vi "CalculateAngle_noDIO_annotated.vi"(8 "dc":dbl, 9 "Robot Beta":dbl, 10 "Robot Alpha":dbl, 11 "Beacon Theta":dbl) -> (0 "Y Position":dbl, 3 "X Position":dbl)   [LabVIEW 2014]
panel:
  out "d1":dbl
  out "K":dbl
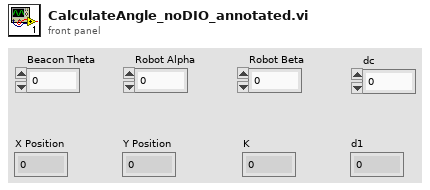
[diagram p1: front panel]
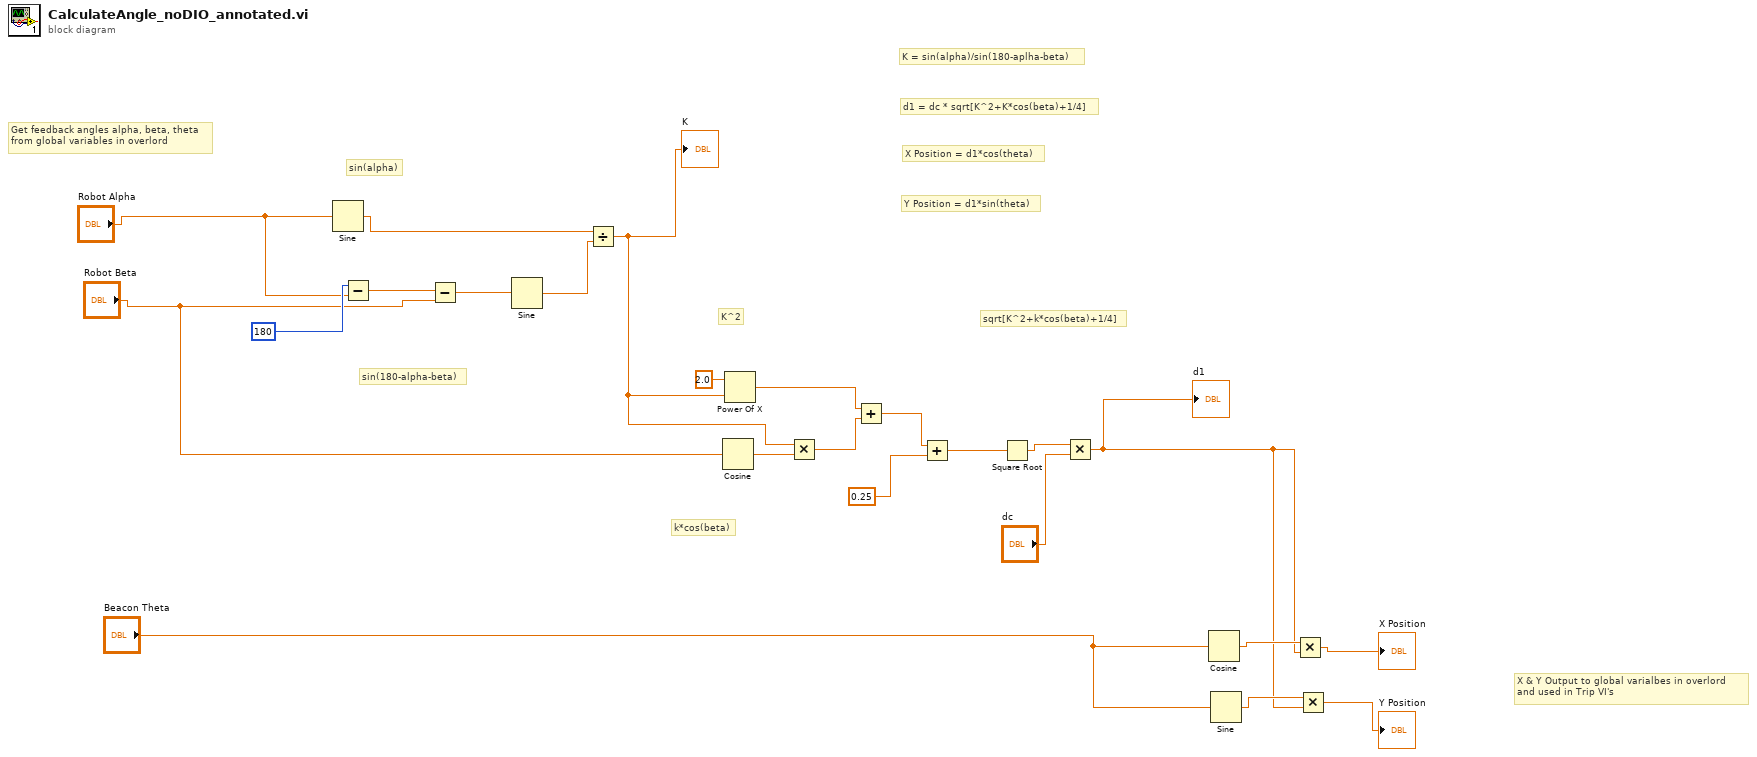
[diagram p0: block diagram]
diagram:
  # "X & Y Output to global varialbes in overlord\nand used in Trip VI's"
  # "Y Position = d1*sin(theta)"
  # "X Position = d1*cos(theta)"
  # "d1 = dc * sqrt[K^2+K*cos(beta)+1/4]"
  # "K = sin(alpha)/sin(180-aplha-beta)"
  # "sqrt[K^2+k*cos(beta)+1/4]"
  # "k*cos(beta)"
  # "K^2"
  # "sin(180-alpha-beta)"
  # "sin(alpha)"
  # "Get feedback angles alpha, beta, theta\nfrom global variables in overlord"
  n1 = Sine(x="Robot Alpha") -> (sin(x)=w19:dbl)
  n2 = Subtract(x=180, y="Robot Alpha") -> (x-y=w21:dbl)
  n3 = Subtract(x=w21, y="Robot Beta") -> (x-y=w20:dbl)
  n4 = Sine(x=w20) -> (sin(x)=w18:dbl)
  n5 = Divide(x=w19, y=w18) -> (x/y=w14:dbl)
  "K" <- w14
  n6 = Cosine(x="Robot Beta") -> (cos(x)=w15:dbl)
  n7 = Power Of X(1:w14, 2:2.0 ("y")) -> (0:w13:dbl)
  n8 = Multiply(x=w14, y=w15) -> (x*y=w12:dbl)
  n9 = Add(x=w13, y=w12) -> (x+y=w11:dbl)
  n10 = Add(x=w11, y=0.25) -> (x+y=w9:dbl)
  n11 = Square Root(x=w9) -> (sqrt(x)=w8:dbl)
  n12 = Multiply(x=w8, y="dc") -> (x*y=w3:dbl)
  "d1" <- w3
  n13 = Cosine(x="Beacon Theta") -> (cos(x)=w5:dbl)
  n14 = Sine(x="Beacon Theta") -> (sin(x)=w4:dbl)
  n15 = Multiply(x=w5, y=w3) -> (x*y=→"X Position":dbl)
  n16 = Multiply(x=w4, y=w3) -> (x*y=→"Y Position":dbl)
